vi "init.vi"(8 "error in (no error)":errorcluster, 11 "ChicagoStyleCheesePizza in":refnum<class "ChicagoStyleCheesePizza.lvclass">) -> (0 "error out":errorcluster, 3 "ChicagoStyleCheesePizza out":refnum<class "ChicagoStyleCheesePizza.lvclass">)   [LabVIEW 2021, in "ChicagoStyleCheesePizza.lvclass"]
uses:
  ChicagoStyleCheesePizza.lvclass
panel:
  # "Connector Pane"
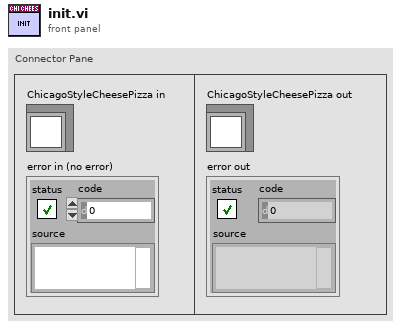
[diagram p1: front panel]
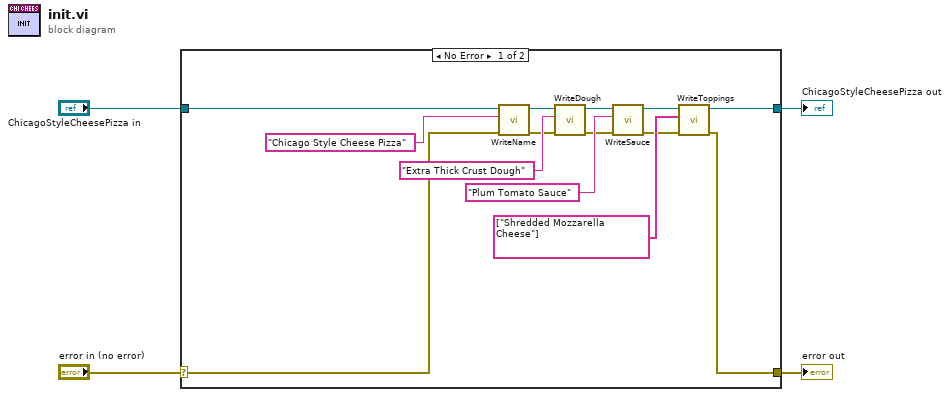
[diagram p0: block diagram]
diagram:
  n1 = case shown="No Error" "error in (no error)" {
    selector: "error in (no error)" -> [w7 w20]
    tunnel: [w8 w20] -> w3
    tunnel: [w5 w19] -> w1
    tunnel: "ChicagoStyleCheesePizza in" -> [w6 w19]
    frame No Error {
      n2 = call-dynamic "WriteName.vi"("error in (no error)"=w7, "name"="Chicago Style Cheese Pizza", "object in"=w6) -> ("error out"=w11:errorcluster, "object out"=w16:refnum<class "ChicagoStyleCheesePizza.lvclass">)  [unwired: 7 in]
      n3 = call-dynamic "WriteDough.vi"("error in (no error)"=w11, "dough"="Extra Thick Crust Dough", "object in"=w16) -> ("error out"=w10:errorcluster, "object out"=w15:refnum<class "ChicagoStyleCheesePizza.lvclass">)  [unwired: 7 in]
      n4 = call-dynamic "WriteSauce.vi"("error in (no error)"=w10, "sauce"="Plum Tomato Sauce", "object in"=w15) -> ("error out"=w9:errorcluster, "object out"=w13:refnum<class "ChicagoStyleCheesePizza.lvclass">)  [unwired: 7 in]
      n5 = call-dynamic "WriteToppings.vi"("error in (no error)"=w9, "toppings"=string[] ["Shredded Mozzarella Cheese"], "object in"=w13) -> ("error out"=w8:errorcluster, "object out"=w5:refnum<class "ChicagoStyleCheesePizza.lvclass">)  [unwired: 7 in]
    }
    frame Error {
    }
  }
  "error out" <- w3
  "ChicagoStyleCheesePizza out" <- w1
